vi "subMFD_FLP Filtering.vi"() -> ()   [LabVIEW 2023]
uses:
  <vilib>/addons/Digital Filter Design/_Objects.llb/DFD Multirate Filter Obj.ctl
  <vilib>/addons/Digital Filter Design/_Objects.llb/DFD Multirate Mode.ctl
  <vilib>/addons/Digital Filter Design/_Objects.llb/DFD Coef Norm Type.ctl
  <vilib>/addons/Digital Filter Design/_Objects.llb/DFD Round-off Mode.ctl
  <vilib>/addons/Digital Filter Design/_Objects.llb/DFD FXP MRate Multiply Mode.ctl
  <vilib>/addons/Digital Filter Design/Multirate.llb/DFD MRate Filtering (Wfm).vi
  <vilib>/measure/maspectr.llb/FFT Spectrum (Mag-Phase) for 1 Chan.vi
  <vilib>/addons/Digital Filter Design/NI_DigFilterLicensed.lvlib
  <vilib>/measure/NI_MABase.lvlib
  <vilib>/measure/NI_MAPro.lvlib
panel:
  in  "Option":enum32{"waveform", "spectrum"}(radio)
  in  "Frequency":dbl=1000.001 min=0.001 max=24000.0 step=1.0 format="%_3p Hz"
  in  "Signal Type":u16(ring) items=["Sine Wave", "Triangle Wave", "Square Wave", "Sawtooth Wave"]
  out "Signals":cluster{"fs [Hz]":dbl, "dt":dbl, "Y":dbl[]}[](graph)
  out "Successful Design?":bool
  out "multirate filter out":T1={"mMRate_Structure"=enum."FIR", "mMRate_Mode"=0, "mMRate_Factor"=-1, "mMRate_FIRParams"={"mMRate_FIR_H"=[], "mMRate_FIR_IsNyquist?"=FALSE, "mMRate_FIR_IsSymmetric?"=FALSE}, "mMRate_CICParams"={"mMRate_CIC_#Stage"=0, "mMRate_CIC_Lag"=1, "mMRate_CIC_Type"=enum."Lowpass"}, "mMRate_Order"=0, "mMRate_Version"="2.0", "mMRate_Comments"="", "mMRate_RationalFactor"={"mMRate_L"=-1, "mMRate_M"=-1}, "mMRate_Fs"=1.0, "mMRate_Quantized?"=FALSE, "mMRate_QFilterGain"=1.0, "mMRate_CoefWl"=16, "mMRate_Scaling"={"mMRate_ScaleByPowerOf2?"=FALSE, "mMRate_ScaleType"=enum."No Norm"}, "mMRate_InputWl"=16, "mMRate_OutputWl"=16, "mMRate_OutputMode"=enum."Truncation", "mMRate_MultMode"=enum."Truncated", "mMRate_BitPruning"=FALSE, "mMRate_GainWl"=16, "mMRate_OutputFwl"=0, "mMRate_SumIwl"=0, "mMRate_InputIwl "=16, "mMRate_SumWl"=32, "mMRate_CoefIwl"=0} {"mMRate_SumWl" min=1 max=32 step=1; "mMRate_InputIwl" min=1 max=32 step=1; "mMRate_GainWl" min=1 max=32 step=1; "mMRate_OutputWl" min=1 max=32 step=1; "mMRate_InputWl" min=1 max=32 step=1; "mMRate_CoefWl" min=1 max=32 step=1; "mMRate_Mode" items=["Default"=-1, "No Rate Change"=0, "Interpolation"=1, "Decimation"=2, "Interpolated"=3, "Rational"=4]}
  in  "multirate filter in":T1={"mMRate_Structure"=enum."FIR", "mMRate_Mode"=0, "mMRate_Factor"=-1, "mMRate_FIRParams"={"mMRate_FIR_H"=[], "mMRate_FIR_IsNyquist?"=FALSE, "mMRate_FIR_IsSymmetric?"=FALSE}, "mMRate_CICParams"={"mMRate_CIC_#Stage"=0, "mMRate_CIC_Lag"=1, "mMRate_CIC_Type"=enum."Lowpass"}, "mMRate_Order"=0, "mMRate_Version"="2.0", "mMRate_Comments"="", "mMRate_RationalFactor"={"mMRate_L"=-1, "mMRate_M"=-1}, "mMRate_Fs"=1.0, "mMRate_Quantized?"=FALSE, "mMRate_QFilterGain"=1.0, "mMRate_CoefWl"=16, "mMRate_Scaling"={"mMRate_ScaleByPowerOf2?"=FALSE, "mMRate_ScaleType"=enum."No Norm"}, "mMRate_InputWl"=16, "mMRate_OutputWl"=16, "mMRate_OutputMode"=enum."Truncation", "mMRate_MultMode"=enum."Truncated", "mMRate_BitPruning"=FALSE, "mMRate_GainWl"=16, "mMRate_OutputFwl"=0, "mMRate_SumIwl"=0, "mMRate_InputIwl "=16, "mMRate_SumWl"=32, "mMRate_CoefIwl"=0} {"mMRate_SumWl" min=1 max=32 step=1; "mMRate_InputIwl" min=1 max=32 step=1; "mMRate_GainWl" min=1 max=32 step=1; "mMRate_OutputWl" min=1 max=32 step=1; "mMRate_InputWl" min=1 max=32 step=1; "mMRate_CoefWl" min=1 max=32 step=1; "mMRate_Mode" items=["Default"=-1, "No Rate Change"=0, "Interpolation"=1, "Decimation"=2, "Interpolated"=3, "Rational"=4]}
  out "OK":bool
  in  "stop":bool
  # "Signals"
  # "Demo Program"
  # "Signal Source"
  # "Options"
  # "Frequency"
  # "Signal Type"
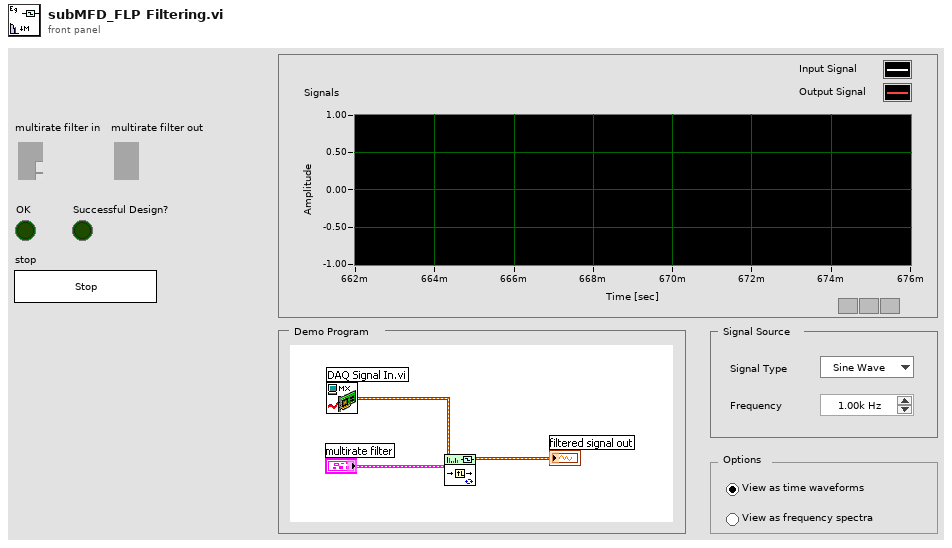
[diagram p1: front panel]
types:
  T1 = typedef "NI_DigFilterLicensed.lvlib/DFD Multirate Filter Obj.ctl" = cluster{"mMRate_Structure":enum16{"CIC", "FIR", "IIR", "Lattice"}, "mMRate_Mode":T2, "mMRate_Factor":i32, "mMRate_FIRParams":cluster{"mMRate_FIR_H":dbl[], "mMRate_FIR_IsNyquist?":bool, "mMRate_FIR_IsSymmetric?":bool}, "mMRate_CICParams":cluster{"mMRate_CIC_#Stage":i32, "mMRate_CIC_Lag":i32, "mMRate_CIC_Type":enum16{"Lowpass", "Highpass"}}, "mMRate_Order":i32, "mMRate_Version":string, "mMRate_Comments":string, "mMRate_RationalFactor":cluster{"mMRate_L":i32, "mMRate_M":i32}, "mMRate_Fs":dbl, "mMRate_Quantized?":bool, "mMRate_QFilterGain":dbl, "mMRate_CoefWl":i16, "mMRate_Scaling":cluster{"mMRate_ScaleByPowerOf2?":bool, "mMRate_ScaleType":T3}, "mMRate_InputWl":i16, "mMRate_OutputWl":i16, "mMRate_OutputMode":T4, "mMRate_MultMode":T5, "mMRate_BitPruning":bool, "mMRate_GainWl":i16, "mMRate_OutputFwl":i16, "mMRate_SumIwl":i16, "mMRate_InputIwl ":i16, "mMRate_SumWl":i16, "mMRate_CoefIwl":i16}
  T2 = typedef "NI_DigFilterLicensed.lvlib/DFD Multirate Mode.ctl" = i16
  T3 = typedef "NI_DigFilterLicensed.lvlib/DFD Coef Norm Type.ctl" = enum16{"No Norm", "Time Domain 1-Norm", "Time Domain 2-Norm", "Time Domain Inf-Norm"}
  T4 = typedef "NI_DigFilterLicensed.lvlib/DFD Round-off Mode.ctl" = enum16{"Nearest", "Truncation"}
  T5 = typedef "NI_DigFilterLicensed.lvlib/DFD FXP MRate Multiply Mode.ctl" = enum16{"Truncated", "Full"}
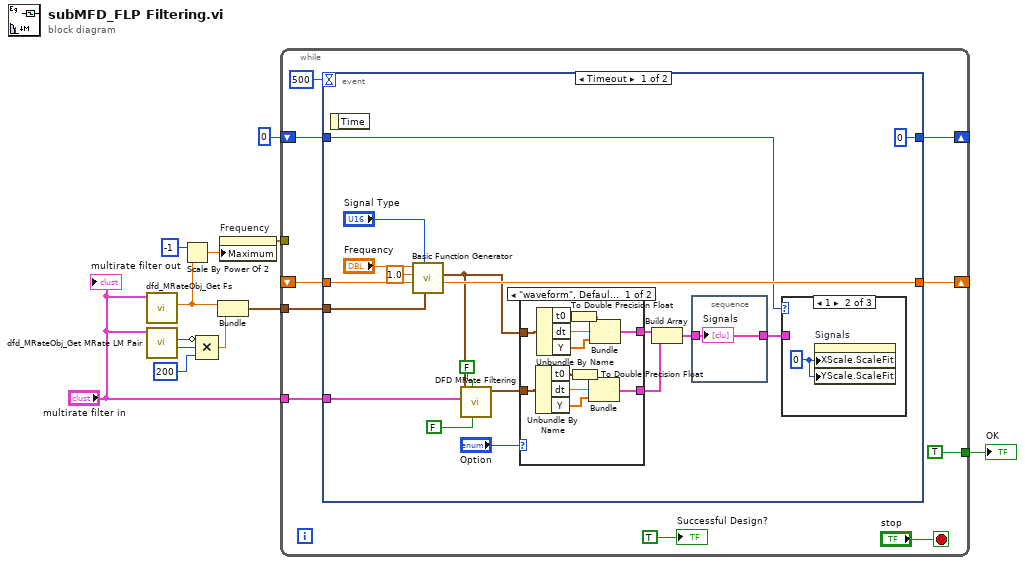
[diagram p0: block diagram]
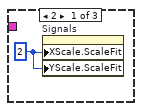
[diagram p2: hidden frame]
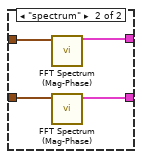
[diagram p4: hidden frame]
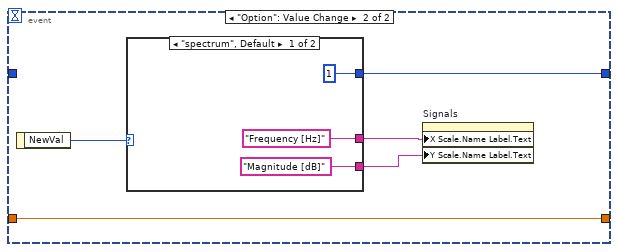
[diagram p5: hidden frame]
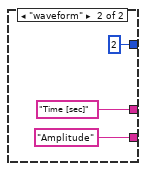
[diagram p6: hidden frame]
diagram:
  n1 = call <vilib>:"dfd_MRateObj_Get Fs.vi"("multirate filter in"="multirate filter in") -> ("fs"=w5:dbl)  [unwired: 10 out]
  n2 = call <vilib>:"dfd_MRateObj_Get MRate LM Pair.vi"("multirate filter in"="multirate filter in") -> ("M"=w9:i32, "L"=w10:i32)  [unwired: 1 in, 8 out]
  n3 = Scale By Power Of 2(n=-1, x=w5) -> (x*2^n=w3:dbl)
  n4 = Compound Arithmetic op=MULTIPLY(invert w10, w9, 200 ("value")) -> (w7:dbl)
  n5 = Bundle("fs"=w5, w7) -> (w6:cluster{"fs":dbl, dbl})  [unwired: 1 out]
  n6 = property on="Frequency" class="DigNum (strict)"("Maximum"=w3) -> (error out=w2:errorcluster)  [unwired: 2 in, 1 out]
  n7 = while {
    tunnel: [TRUE] -> w12
    tunnel: "multirate filter in" -> [w15]
    shift-right: [w17] -> _
    shift-left: _ -> [w18]
    tunnel: w6 -> [w16]
    tunnel: w2 -> [_]
    shift-right: [w13] -> _
    shift-left: 0 -> [w14]
    stop <- "stop" stop-if-true
    n8 = event shown="[0] Timeout" {
      selector: _ -> [_ _]
      dyn-events: _ -> [_ _]
      timeout: 500 -> [_ _]
      tunnel: w18 -> [w37 w64]
      tunnel: [w36 w64] -> w17
      tunnel: w16 -> [w35 _]
      tunnel: w15 -> [w33 _]
      tunnel: w14 -> [w24 _]
      tunnel: [0 w60] -> w13
      event Timeout {
        n9 = event-data() -> ()  [unwired: 2 out]
        n10 = call <vilib>:"Basic Function Generator.vi"("sampling info"=w35, "signal type"="Signal Type", "phase"=w37, "amplitude"=1.0, "frequency"="Frequency") -> ("phase out"=w36:dbl, "signal out"=w32:waveform(dbl))  [unwired: 4 in, 1 out]
        n11 = call-poly <vilib>:"DFD MRate Filtering.vi"("zero phase? (T)"=FALSE, "init? (F)"=FALSE, "multirate filter"=w33, "signal in"=w32) -> ("signal out"=w31:waveform(dbl))  [unwired: 1 in, 6 out]
        n12 = case shown="\"waveform\", Default" "Option" {
          tunnel: w32 -> [w55 w59]
          tunnel: w31 -> [w54 w56]
          tunnel: [w51 w57] -> w30
          tunnel: [w50 w58] -> w29
          frame "waveform", Default {
            n13 = Unbundle By Name(w54) -> ("t0"=w45:timestamp, "dt"=w49:dbl, "Y"=w48:dbl[])
            n14 = Unbundle By Name(w55) -> ("t0"=w47:timestamp, "dt"=w53:dbl, "Y"=w52:dbl[])
            n15 = To Double Precision Float(number=w47) -> (double precision float=w46:dbl)
            n16 = To Double Precision Float(number=w45) -> (double precision float=w44:dbl)
            n17 = Bundle(w44, "dt"=w49, "Y"=w48) -> (w50:cluster{dbl, "dt":dbl, "Y":dbl[]})  [unwired: 1 out]
            n18 = Bundle(w46, "dt"=w53, "Y"=w52) -> (w51:cluster{dbl, "dt":dbl, "Y":dbl[]})  [unwired: 1 out]
          }
          frame "spectrum" {
            n19 = call-poly <vilib>:"FFT Spectrum (Mag-Phase).vi"("time signal"=w59) -> ("magnitude"=w57:cluster{"f0":dbl, "df":dbl, "magnitude":dbl[]})  [unwired: 6 in, 4 out]
            n20 = call-poly <vilib>:"FFT Spectrum (Mag-Phase).vi"("time signal"=w56) -> ("magnitude"=w58:cluster{"f0":dbl, "df":dbl, "magnitude":dbl[]})  [unwired: 6 in, 4 out]
          }
        }
        n21 = Build Array(w30, w29) -> (w28:cluster{"f0":dbl, "df":dbl, "magnitude":dbl[]}[])
        n22 = stacked-sequence {
          tunnel: w28 -> [w43]
          tunnel: [w43] -> w23
          frame #0 {
            "Signals" <- w43
          }
        }
        n23 = case shown="1" w24 {
          tunnel: w23 -> [_ _ _]
          frame 2 {
            w41 = u8 2 ("X Scale.Scale Fit")
            n24 = property on="Signals" class="WFGraph (strict)"("XScale.ScaleFit"=w41, "YScale.ScaleFit"=w41) -> ()  [unwired: 2 in, 2 out]
          }
          frame 1 {
            w42 = u8 0 ("X Scale.Scale Fit")
            n25 = property on="Signals" class="WFGraph (strict)"("XScale.ScaleFit"=w42, "YScale.ScaleFit"=w42) -> ()  [unwired: 2 in, 2 out]
          }
          frame 0, Default {
          }
        }
      }
      event "Option": Value Change {
        n26 = event-data() -> ("NewVal"=w63:enum32{"waveform", "spectrum"})  [unwired: 1 out]
        n27 = case shown="\"spectrum\", Default" w63 {
          tunnel: ["Frequency [Hz]" "Time [sec]"] -> w62
          tunnel: ["Magnitude [dB]" "Amplitude"] -> w61
          tunnel: [1 2] -> w60
          frame "spectrum", Default {
          }
          frame "waveform" {
          }
        }
        n28 = property on="Signals" class="WFGraph (strict)"("X Scale.Name Label.Text"=w62, "Y Scale.Name Label.Text"=w61) -> ()  [unwired: 2 in, 2 out]
      }
    }
    "Successful Design?" <- TRUE ("Successful Design?")
  }
  "OK" <- w12
  "multirate filter out" <- "multirate filter in"
